vi "Launch Tag Watchlist UI.vi"(8 "error in (no error)":errorcluster, 10 "Shutdown Event":refnum<user-event>) -> (0 "error out":errorcluster)   [LabVIEW 2018, in "Tag Watchlist.lvlib"]
doc: "Tag watchlist launcher. Allows non-blocking launch of Tag Watchlist window (fire and forget), while allowing only one instance to be running.\n\nThe input Shutdown Event should be used to shutdown the Tag Watchlist window in the event of main application shutdown."
uses:
  Tag Watchlist.lvlib
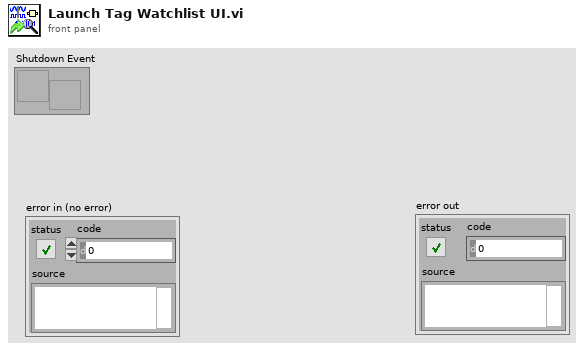
[diagram p1: front panel]
types:
  T1 = enum32{"Bad", "Idle", "Run top level", "Running"}
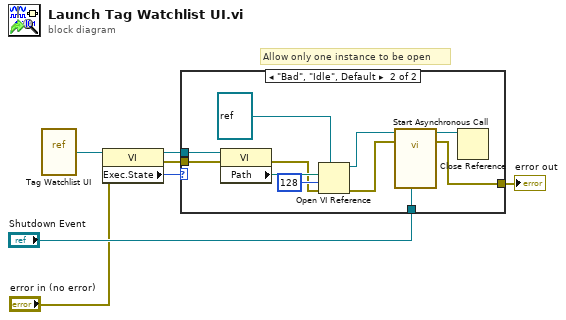
[diagram p0: block diagram]
diagram:
  # "Allow only one instance to be open"
  n1 = vi-ref "Tag Watchlist UI.vi"() -> (w7:refnum<vi>)
  n2 = property class="VI"(reference=w7, error in="error in (no error)") -> (reference out=w5:refnum<vi>, error out=w4:errorcluster, "Exec.State"=w6:T1)
  n3 = case shown="\"Bad\", \"Idle\", Default" w6 {
    tunnel: w5 -> [_ w19]
    tunnel: w4 -> [w8 w18]
    tunnel: "Shutdown Event" -> [_ w11]
    tunnel: [w8 w9] -> w2
    frame "Run top level", "Running" {
    }
    frame "Bad", "Idle", Default {
      n4 = property class="VI"(reference=w19, error in=w18) -> (error out=w14:errorcluster, "Path"=w17:path)  [unwired: 1 out]
      n5 = Open VI Reference(type specifier VI Refnum (for type only)=refnum<vi> refnum, vi path=w17, options=128, error in (no error)=w14) -> (vi reference=w12:refnum<vi>, error out=w13:errorcluster)  [unwired: 2 in]
      n6 = call-by-ref "Start Asynchronous Call"(reference=w12, error in=w13, "Shutdown Event"=w11) -> (reference out=w10:refnum<vi>, error out=w9:errorcluster)  [unwired: 11 in]
      n7 = Close Reference(reference=w10) -> ()  [unwired: 1 in, 1 out]
    }
  }
  "error out" <- w2
